vi "Get RemIO Read Scaling Factor.vi"(8 "error in (no error)":errorcluster, 10 "11100 in":refnum<class "11100.lvclass">, 11 "Node Ptr In":T1 format="%.0x") -> (0 "error out":errorcluster, 1 "Scaling Factors":dbl[](array[numeric]), 2 "11100 out":refnum<class "11100.lvclass">, 3 "Node Ptr Out":T1 format="%.0x", 5 "Per Channel?":bool)   [LabVIEW 2017, in "Modules.lvlib" / "11100.lvclass"]
doc: "This VI Returns the scaling factors for REM IO Input Modules"
uses:
  11100.lvclass
  <vilib>/NI Veristand/Custom Device API/Custom Device Item Ref.ctl
  11100.lvclass/11100.ctl
  06eeaf79-0fb5-4458-8616-2d8867bb1cb7.vi
  RemIO Module/Get RemIO Library Path.vi
  <vilib>/NI Veristand/Custom Device API/Custom Device API.lvlib
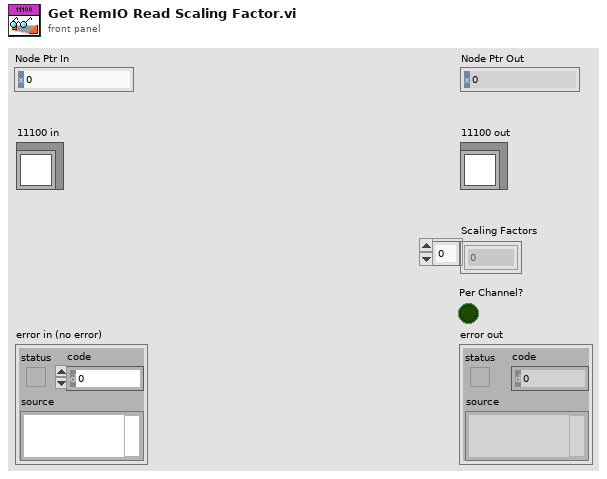
[diagram p1: front panel]
types:
  T1 = typedef "Custom Device API.lvlib/Custom Device Item Ref.ctl" = u64
  T2 = typedef "NI ECAT Remote IO.lvlib/channel number REM-11100.ctl" = u8
  T3 = typedef "NI ECAT Remote IO.lvlib/input filter time REM-11100.ctl" = u8
  T4 = typedef "NI ECAT Remote IO.lvlib/mean-value REM-11100.ctl" = u8
  T5 = typedef "NI ECAT Remote IO.lvlib/measuring range REM-11100.ctl" = u8
  T6 = cluster{"channel number":T2, "input filter time":T3, "mean-value":T4, "measuring range":T5}[]
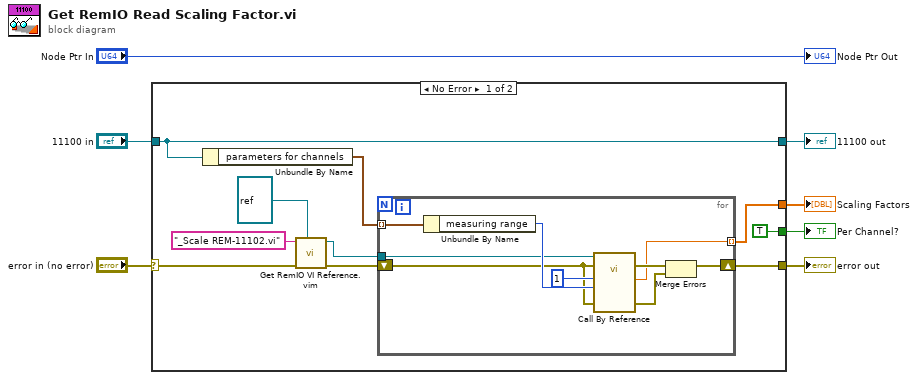
[diagram p0: block diagram]
diagram:
  n1 = case shown="No Error" "error in (no error)" {
    selector: "error in (no error)" -> [w12 w28]
    tunnel: [w16 w28] -> w3
    tunnel: [w14 w27] -> w2
    tunnel: "11100 in" -> [w14 w27]
    tunnel: [w15 _] -> w4
    tunnel: [TRUE _] -> w5
    frame No Error {
      n2 = Unbundle By Name(w14) -> ("parameters for channels"=w13:T6)
      n3 = call "Get RemIO VI Reference.vim"("name or relative path"="_Scale REM-11102.vi", "error in (no error)"=w12, "type specifier VI Refnum (for type only)"=refnum<vi> refnum) -> ("vi reference"=w8:refnum<vi>, "error out"=w11:errorcluster)  [unwired: 6 in]
      n4 = for {
        shift-right: [w19] -> w16
        shift-left: w11 -> [w20]
        tunnel: [w23] -> w15 mode=indexing
        tunnel: w13 -> [w26] mode=indexing
        tunnel: w8 -> [w18]
        n5 = Unbundle By Name(w26) -> ("measuring range"=w21:T5)
        n6 = call-by-ref "?"(reference=w18, error in=w20, 8:"error in (no error)"=w20, "measuring range"=w21, "raw data"=u16 1) -> (error out=w24:errorcluster, 0:"error out"=w25:errorcluster, "scaled data"=w23:dbl)  [unwired: 7 in, 1 out]
        n7 = Merge Errors(w24, w25) -> (w19:errorcluster)
      }
    }
    frame Error {
    }
  }
  "error out" <- w3
  "11100 out" <- w2
  "Scaling Factors" <- w4
  "Per Channel?" <- w5
  "Node Ptr Out" <- "Node Ptr In"
